vi "Test.vi"() -> ()   [LabVIEW 2013]
uses:
  <instrlib>/HadCon/HadCon.lvlib
panel:
  out "Help":string
  out "Error Out":errorcluster
  in  "VISA resource name":refnum<visa-resource-name>
  out "Instrument Firmware Revision":string
  out "Instrument Driver Revision":string
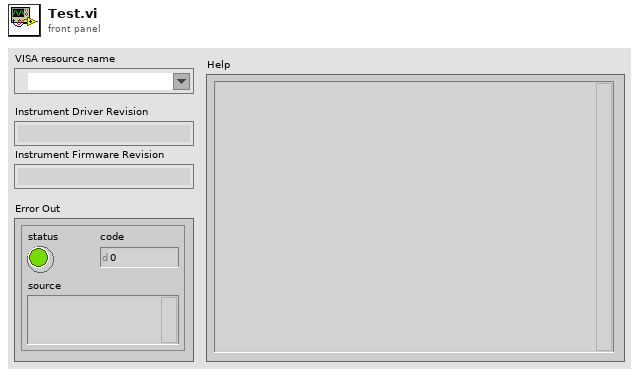
[diagram p1: front panel]
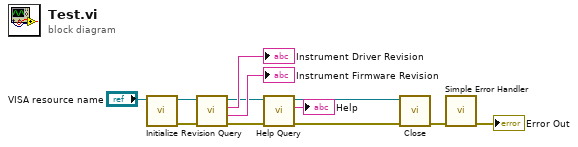
[diagram p0: block diagram]
diagram:
  n1 = call <instrlib>:"Initialize.vi"("VISA resource name"="VISA resource name") -> ("error out"=w11:errorcluster, "VISA resource name out"=w12:refnum<visa-resource-name>)  [unwired: 9 in]
  n2 = call <instrlib>:"Revision Query.vi"("error in (no error)"=w11, "VISA resource name"=w12) -> ("error out"=w4:errorcluster, "Instrument Firmware Revision"=→"Instrument Firmware Revision":string, "Instrument Driver Revision"=→"Instrument Driver Revision":string, "VISA resource name out"=w5:refnum<visa-resource-name>)  [unwired: 6 in]
  n3 = call <instrlib>:"Help Query.vi"("error in (no error)"=w4, "VISA resource name"=w5) -> ("error out"=w2:errorcluster, "Help"=→"Help":string, "VISA resource name out"=w3:refnum<visa-resource-name>)  [unwired: 7 in]
  n4 = call <instrlib>:"Close.vi"("error in (no error)"=w2, "VISA resource name"=w3) -> ("error out"=w8:errorcluster)  [unwired: 9 in]
  n5 = call <vilib>:"Simple Error Handler.vi"("error in (no error)"=w8) -> ("error out"=→"Error Out":errorcluster)  [unwired: 4 in, 4 out]
